vi "Intake_Ball_Execute.vi"() -> ()   [LabVIEW 2018]
uses:
  <vilib>/Rock Robotics/WPI/ThirdParty/Phoenix-LabVIEW/Motor Controller/Controls/CTRE_Phoenix_MotorControl_ControlMode.ctl
  <vilib>/Rock Robotics/WPI/DriverStation/WPI_DriverStationRobotMode2.ctl
  Global_Variables/Intake_Ball_Globals.vi
  Global_Variables/Robot_Global_Data.vi
  Global_Variables/Sensor_Values.vi
panel:
  in  "Ball_Leaving":dbl=1.0
  in  "Stall":dbl=0.15
  in  "Out_Speed":dbl=-0.85
  in  "In_Speed":dbl=1.0
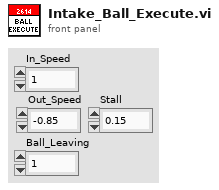
[diagram p1: front panel]
types:
  T1 = typedef "WPI_MotorControlDeviceRef.ctl" = cluster{"DeviceStatus":errorcluster, "Type":T2, "PWM":cluster{"PWM Channel":T3, "DeadBand":T4}, "CAN":cluster{"Device Number":u8, "SetOutput VI Ref":variant, "GetOutput VI Ref":variant, "Enable VI Ref":variant, "Disable VI Ref":variant, "Data":variant}, "Invert":bool, "DIO PWM":cluster{"PWM \"Enable\" Channel":T3, "DIOChannel":T5, "PWM Rate":dbl}}
  T2 = typedef "WPI_MotorControlType.ctl" = enum16{"PWM", "CAN", "DIO PWM"}
  T3 = typedef "FPGA_DIOPWMChannel.ctl" = enum8{"PWM 0", "PWM 1", "PWM 2", "PWM 3", "PWM 4", "PWM 5", "PWM 6", "PWM 7", "PWM 8", "PWM 9", "PWM MXP 0", "PWM MXP 1", "PWM MXP 2", "PWM MXP 3", "PWM MXP 4", "PWM MXP 5", "PWM MXP 6", "PWM MXP 7", "PWM MXP 8", "PWM MXP 9", "Invalid"}
  T4 = typedef "WPI_PWMDeadband.ctl" = cluster{"Name":string, "maxPositivePwm":i32, "minPositivePwm":i32, "centerPwm":i32, "maxNegativePwm":i32, "minNegativePwm":i32, "angularRange":u16}
  T5 = typedef "FPGA_DIOChannel.ctl" = enum8{"DIO 0", "DIO 1", "DIO 2", "DIO 3", "DIO 4", "DIO 5", "DIO 6", "DIO 7", "DIO 8", "DIO 9", "DIO MXP 0", "DIO MXP 1", "DIO MXP 2", "DIO MXP 3", "DIO MXP 4", "DIO MXP 5", "DIO MXP 6", "DIO MXP 7", "DIO MXP 8", "DIO MXP 9", "DIO MXP 10", "DIO MXP 11", "DIO MXP 12", "DIO MXP 13", "DIO MXP 14", "DIO MXP 15", "SPI Port CS1", "SPI Port CS2", "SPI Port CS3", "SPI Port MISO", "SPI Port MOSI", "Invalid"}
  T6 = typedef "WPI_DriverStationRobotMode2.ctl" = enum16{"Autonomous Disabled", "Autonomous Enabled", "Teleop Disabled", "Teleop Enabled", "Disconnected", "Finish", "Test Disabled", "Test Enabled", "Emergency Stopped"}
  T7 = typedef "Intake_Ball_Notifier.ctl" = cluster{"Intake_Ball_Control_Type":T8, "Manual_In":bool, "Manual_Out":bool, "Ball_In":bool, "Ball_Out":bool, "Parameter_One":dbl, "Parameter_Two":dbl, "Parameter_Three":dbl, "Step":i32, "Ball_Notifier":refnum<notifier>}
  T8 = typedef "Intake_Ball_Control_Type.ctl" = enum16{"No_Op", "Manual_In", "Manual_Out", "In_Sensor_Stop", "Out_Teleop", "Out", "Stall"}
  T9 = typedef "CTRE_Phoenix_MotorControl_ControlMode.ctl" = u16
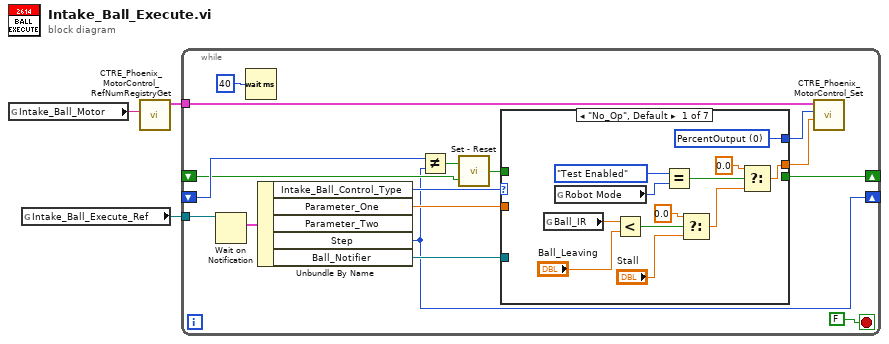
[diagram p0: block diagram]
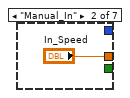
[diagram p2: hidden frame]
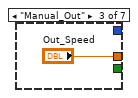
[diagram p3: hidden frame]
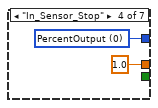
[diagram p4: hidden frame]
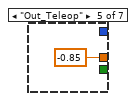
[diagram p5: hidden frame]
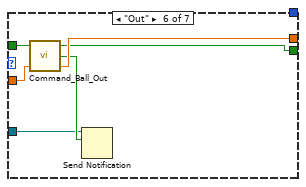
[diagram p6: hidden frame]
diagram:
  n1 = global read "Intake_Ball_Globals.vi" "Intake_Ball_Motor"() -> (w1:string)
  n2 = global read "Intake_Ball_Globals.vi" "Intake_Ball_Execute_Ref"() -> (w2:refnum<notifier>)
  n3 = call <vilib>:"CTRE_Phoenix_MotorControl_RefNumRegistryGet.vi"("refnum name"=w1) -> ("PhoenixMotorControlDevRef"=w3:T1)  [unwired: 9 in, 1 out]
  n4 = while {
    tunnel: w3 -> [w15]
    tunnel: w2 -> [w12]
    shift-right: [w9] -> _
    shift-left: _ -> [w6]
    shift-right: [w5] -> _
    shift-left: _ -> [w8]
    stop <- FALSE stop-if-true
    n5 = Wait on Notification(notifier=w12) -> (notification=w17:T7)  [unwired: 3 in, 3 out]
    n6 = Wait (ms)(milliseconds to wait=u32 40) -> ()  [unwired: 1 out]
    n7 = Unbundle By Name(w17) -> ("Intake_Ball_Control_Type"=w16:T8, "Parameter_One"=w11:dbl, "Step"=w5:i32, "Ball_Notifier"=w10:refnum<notifier>)  [unwired: 1 out]
    n8 = Not Equal?(x=w8, y=w5) -> (x != y?=w7:bool)
    n9 = call "Set - Reset.vi"("Reset"=w6, "Set"=w7) -> ("Output"=w4:bool)
    n10 = case shown="\"No_Op\", Default" w16 {
      tunnel: [w31 _ _ w35 _ _ _] -> w14
      tunnel: [w25 "In_Speed" "Out_Speed" 1.0 ("f") -0.85 ("f") w41 _] -> w13
      tunnel: w11 -> [_ _ _ _ _ w42 _]
      tunnel: w10 -> [_ _ _ _ _ w38 _]
      tunnel: [_ _ _ _ _ w40 _] -> w9
      tunnel: w4 -> [_ _ _ _ _ w37 _]
      frame "No_Op", Default {
        w31 = T9 0 items=["PercentOutput"=0, "Position"=1, "Velocity"=2, "Current"=3, "Follower"=5, "MotionProfile"=6, "MotionMagic"=7, "MotionProfileArc"=10, "Disabled"=15] ("Control Mode")
        n11 = global read "Sensor_Values.vi" "Ball_IR"() -> (w22:dbl)
        n12 = global read "Robot_Global_Data.vi" "Robot Mode"() -> (w30:T6)
        n13 = Less?(x=w22, y="Ball_Leaving") -> (x < y?=w21:bool)
        n14 = Equal?(x=WPI_DriverStationRobotMode2."Test Enabled", y=w30) -> (x = y?=w28:bool)
        n15 = Select(t=0.0, s=w21, f="Stall") -> (s? t:f=w26:dbl)
        n16 = Select(t=0.0, s=w28, f=w26) -> (s? t:f=w25:dbl)
      }
      frame "Manual_In" {
      }
      frame "Manual_Out" {
      }
      frame "In_Sensor_Stop" {
        w35 = T9 0 items=["PercentOutput"=0, "Position"=1, "Velocity"=2, "Current"=3, "Follower"=5, "MotionProfile"=6, "MotionMagic"=7, "MotionProfileArc"=10, "Disabled"=15] ("Control Mode")
      }
      frame "Out_Teleop" {
      }
      frame "Out" {
        n17 = call "Command_Ball_Out.vi"("Timeout"=w42, "Startup"=w37) -> ("Speed"=w41:dbl, "Completed"=w39:bool, "Reinit"=w40:bool)  [unwired: 1 in]
        n18 = Send Notification(notification=w39, notifier=w38) -> ()  [unwired: 1 in, 2 out]
      }
      frame "Stall" {
      }
    }
    n19 = call <vilib>:"CTRE_Phoenix_MotorControl_Set.vi"("Output"=w13, "Control Mode"=w14, "PhoenixMotorControlDevRef"=w15) -> ()  [unwired: 7 in, 2 out]
  }
